vi "act-0021-1-cor.vi"() -> ()   [LabVIEW 2010]
uses:
  support/c_pi_wilson.ctl
  support/c_pi_penalite.ctl
  support/lv_07.lvlib
panel:
  in  "Pénalité (e)":T1
  in  "Pièce e":T2
  out "error out":errorcluster caption="err out"
  in  "err in":errorcluster
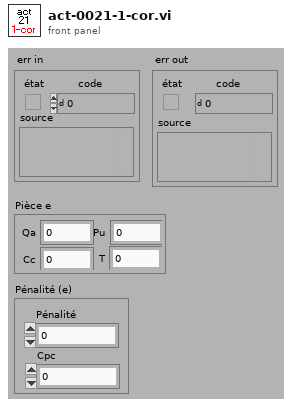
[diagram p1: front panel]
types:
  T1 = typedef "lv_07.lvlib/c_pi_penalite.ctl" = cluster{"Pénalité":dbl, "Cpc":dbl}
  T2 = typedef "lv_07.lvlib/c_pi_wilson.ctl" = cluster{"T":dbl, "Pu":dbl, "Qa":dbl, "Cc":dbl}
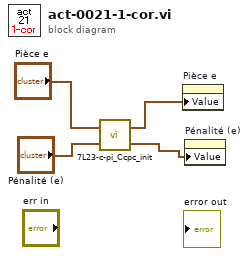
[diagram p0: block diagram]
diagram:
  n1 = call "7L23-c-pi_Ccpc_init.vi"("Pénalité (e)"="Pénalité (e)", "Pièce e"="Pièce e") -> ("Pénalité (s)"=w1:T1, "Pièce s"=w2:T2)
  n2 = property on="Pièce e" class="Clust (strict)"("Value"=w2) -> ()  [unwired: 2 in, 2 out]
  n3 = property on="Pénalité (e)" class="Clust (strict)"("Value"=w1) -> ()  [unwired: 2 in, 2 out]
